vi "presets dialog.vi"(11 "Cluster in":T1={"Country 1 index"=201, "Country 2 index"=0, "countries"=[], "Data"=0, "Curve fit all data"=TRUE, "Curve 1 type"=enum."Exponential", "Curve 2 type"=enum."Exponential", "absolute?"=TRUE, "cursor 1 "=0.0, "cursor 2 "=0.0, "threshold cases"=1} {"Data" items=["cumulative cases", "new cases per day", "deaths"]}) -> (2 "Load?":bool, 3 "Cluster out":T1={"Country 1 index"=201, "Country 2 index"=0, "countries"=[], "Data"=0, "Curve fit all data"=TRUE, "Curve 1 type"=enum."Exponential", "Curve 2 type"=enum."Exponential", "absolute?"=TRUE, "cursor 1 "=0.0, "cursor 2 "=0.0, "threshold cases"=1} {"Data" items=["cumulative cases", "new cases per day", "deaths"]})   [LabVIEW 2019]
uses:
  <vilib>/Utility/sysdir.llb/System Directory Type.ctl
  <vilib>/Utility/config.llb/Write Key (I32).vi
  <vilib>/Utility/config.llb/Write Key (Boolean).vi
  <vilib>/Utility/config.llb/Write Key (Double).vi
  <vilib>/Utility/config.llb/Read Key (I32).vi
  <vilib>/Utility/config.llb/Read Key (Boolean).vi
  <vilib>/Utility/config.llb/Read Key (Double).vi
  <vilib>/Utility/config.llb/NI_LVConfig.lvlib
panel:
  in  "Delete":bool
  in  "Load":bool
  in  "Save Button":bool
  in  "Cancel Button":bool
  in  "Presets":i32(listbox)
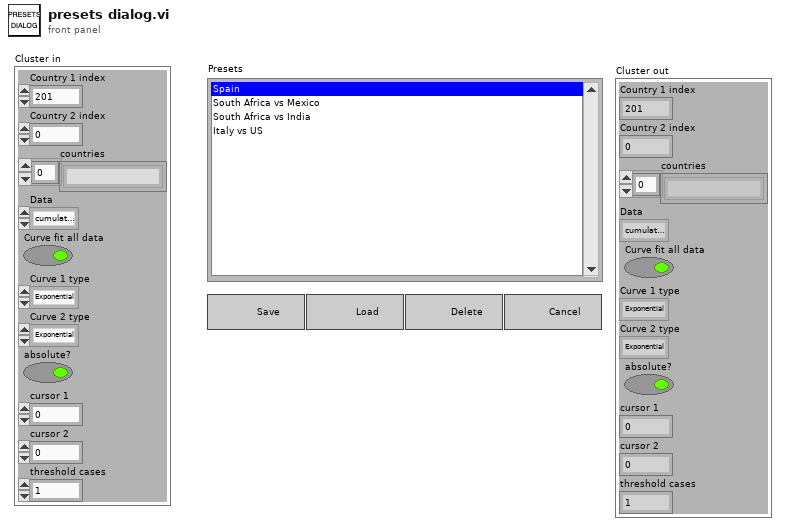
[diagram p1: front panel]
types:
  T1 = cluster{"Country 1 index":i32, "Country 2 index":i32, "countries":string[], "Data":u16, "Curve fit all data":bool, "Curve 1 type":enum16{"Exponential", "Logarithm", "No curve"}, "Curve 2 type":enum16{"Exponential", "Logarithm", "No curve"}, "absolute?":bool, "cursor 1 ":dbl, "cursor 2 ":dbl, "threshold cases":u32}
  T2 = typedef "System Directory Type.ctl" = i32
  T3 = typedef "NI_LVConfig.lvlib/Config Data RefNum.ctl" = refnum<k1>
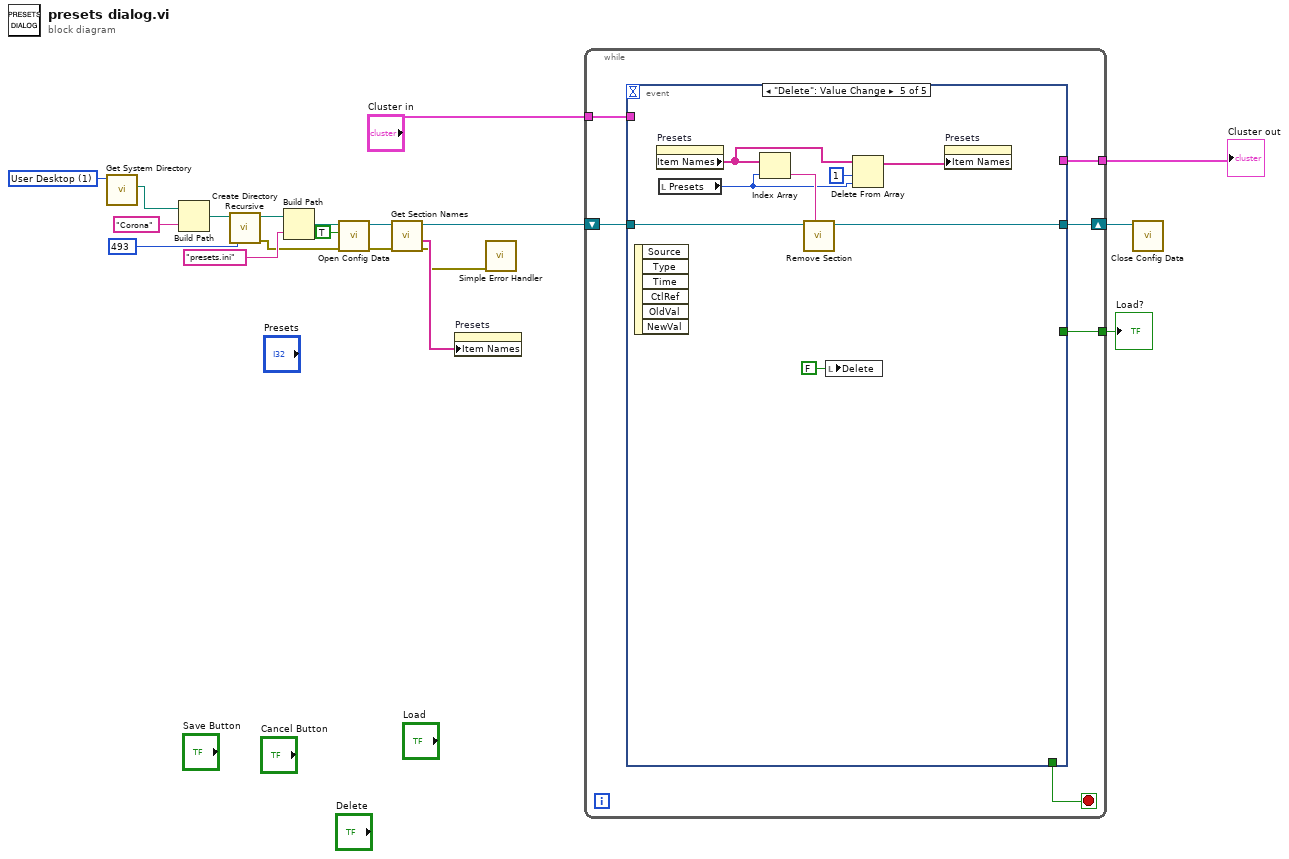
[diagram p0: block diagram]
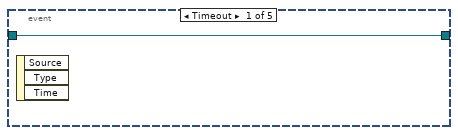
[diagram p2: hidden frame]
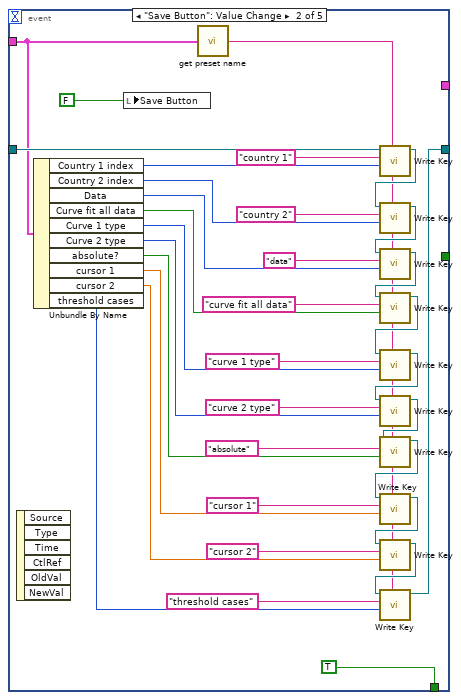
[diagram p3: hidden frame]
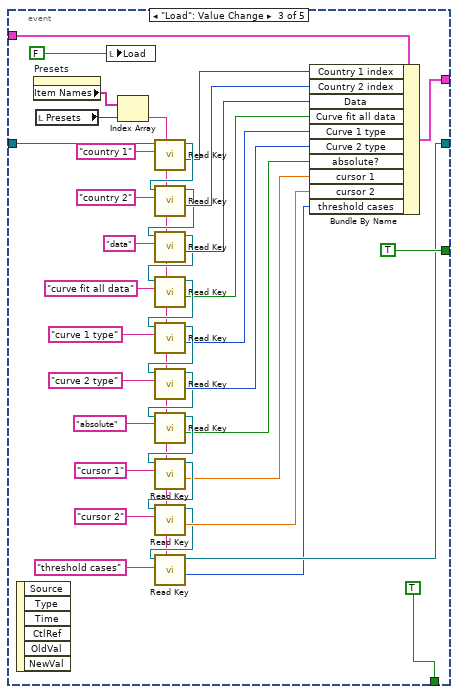
[diagram p4: hidden frame]
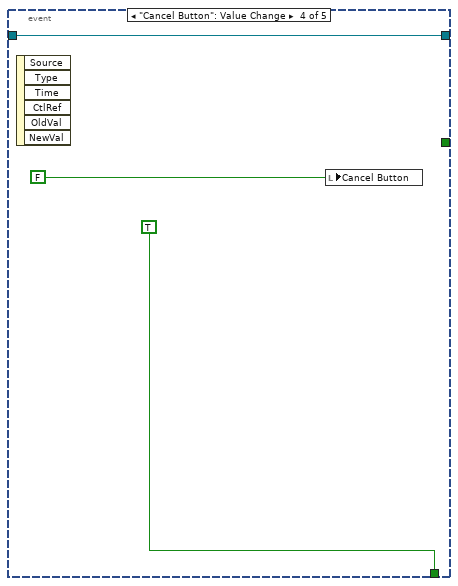
[diagram p5: hidden frame]
diagram:
  w19 = T2 1 items=["User Home"=0, "User Desktop"=1, "User Documents"=2, "User Application Data"=3, "User Preferences"=4, "User Temporary"=5, "Public Documents"=6, "Public Application Data"=7, "Public Preferences"=8, "Public Cache"=13, "System Core Libraries"=9, "System Installed Libraries"=10, "Application Files"=11, "Boot Volume Root"=12] ("system directory type")
  n1 = call <vilib>:"Get System Directory.vi"("system directory type"=w19) -> ("system directory"=w18:path)  [unwired: 10 in]
  n2 = Build Path(base path=w18, name or relative path="Corona") -> (appended path=w7:path)
  n3 = call <vilib>:"Create Directory Recursive.vi"("permissions"=i16 493, "directory"=w7) -> ("error out"=w5:errorcluster, "directory copy"=w6:path)  [unwired: 3 in, 1 out]
  n4 = Build Path(base path=w6, name or relative path="presets.ini") -> (appended path=w15:path)
  n5 = call <vilib>:"Open Config Data.vi"("error in (no error)"=w5, "create file if necessary (T)"=TRUE, "configuration file path"=w15) -> ("error out"=w9:errorcluster, "refnum"=w13:T3)  [unwired: 6 in, 1 out]
  n6 = call <vilib>:"Get Section Names.vi"("error in (no error)"=w9, "refnum"=w13) -> ("error out"=w8:errorcluster, "section names"=w11:string[], "refnum out"=w12:T3)  [unwired: 7 in]
  n7 = property on="Presets" class="LstBox (strict)"("Item Names"=w11) -> ()  [unwired: 2 in, 2 out]
  n8 = call <vilib>:"Simple Error Handler.vi"("error in (no error)"=w8) -> ()  [unwired: 4 in, 5 out]
  n9 = while {
    shift-right: [w24] -> w10
    shift-left: w12 -> [w25]
    tunnel: "Cluster in" -> [w22]
    tunnel: [w21] -> w1
    tunnel: [w20] -> w3
    stop <- w23 stop-if-true
    n10 = event shown="[4] \"Delete\": Value Change" {
      selector: _ -> [_ _ _ _ _]
      dyn-events: _ -> [_ _ _ _ _]
      timeout: _ -> [_ _ _ _ _]
      tunnel: w25 -> [w26 w61 w100 w102 w111]
      tunnel: [w26 w31 w66 w102 w109] -> w24
      tunnel: [_ TRUE TRUE TRUE _] -> w23
      tunnel: w22 -> [_ w53 w92 _ _]
      tunnel: [_ _ w91 _ _] -> w21
      tunnel: [_ _ TRUE _ _] -> w20
      event Timeout {
        n11 = event-data() -> ()  [unwired: 1 in, 3 out]
      }
      event "Save Button": Value Change {
        n12 = event-data() -> ()  [unwired: 1 in, 6 out]
        n13 = Unbundle By Name(w53) -> ("Country 1 index"=w55:i32, "Country 2 index"=w54:i32, "Data"=w51:u16, "Curve fit all data"=w37:bool, "Curve 1 type"=w36:enum16{"Exponential", "Logarithm", "No curve"}, "Curve 2 type"=w35:enum16{"Exponential", "Logarithm", "No curve"}, "absolute?"=w34:bool, "cursor 1"=w33:dbl, "cursor 2"=w32:dbl, "threshold cases"=w29:u32)
        n14 = local write "Save Button"(FALSE ("Save Button")) -> ()
        n15 = call "get preset name.vi"("Cluster in"=w53) -> ("Preset name out"=w27:string)
        n16 = call-poly <vilib>:"Write Key.vi"("section"=w27, "value"=w55, "key"="country 1", "refnum"=w61) -> ("refnum out"=w57:T3)  [unwired: 5 in, 2 out]
        n17 = call-poly <vilib>:"Write Key.vi"("section"=w27, "value"=w54, "key"="country 2", "refnum"=w57) -> ("refnum out"=w50:T3)  [unwired: 5 in, 2 out]
        n18 = call-poly <vilib>:"Write Key.vi"("section"=w27, "value"=w51, "key"="data", "refnum"=w50) -> ("refnum out"=w49:T3)  [unwired: 5 in, 2 out]
        n19 = call-poly <vilib>:"Write Key.vi"("section"=w27, "value"=w37, "key"="curve fit all data", "refnum"=w49) -> ("refnum out"=w48:T3)  [unwired: 5 in, 2 out]
        n20 = call-poly <vilib>:"Write Key.vi"("section"=w27, "value"=w36, "key"="curve 1 type", "refnum"=w48) -> ("refnum out"=w47:T3)  [unwired: 5 in, 2 out]
        n21 = call-poly <vilib>:"Write Key.vi"("section"=w27, "value"=w35, "key"="curve 2 type", "refnum"=w47) -> ("refnum out"=w46:T3)  [unwired: 5 in, 2 out]
        n22 = call-poly <vilib>:"Write Key.vi"("section"=w27, "value"=w34, "key"="absolute", "refnum"=w46) -> ("refnum out"=w45:T3)  [unwired: 5 in, 2 out]
        n23 = call-poly <vilib>:"Write Key.vi"("section"=w27, "value"=w33, "key"="cursor 1", "refnum"=w45) -> ("refnum out"=w44:T3)  [unwired: 5 in, 2 out]
        n24 = call-poly <vilib>:"Write Key.vi"("section"=w27, "value"=w32, "key"="cursor 2", "refnum"=w44) -> ("refnum out"=w30:T3)  [unwired: 5 in, 2 out]
        n25 = call-poly <vilib>:"Write Key.vi"("section"=w27, "value"=w29, "key"="threshold cases", "refnum"=w30) -> ("refnum out"=w31:T3)  [unwired: 5 in, 2 out]
      }
      event "Load": Value Change {
        n26 = event-data() -> ()  [unwired: 1 in, 6 out]
        n27 = property on="Presets" class="LstBox (strict)"() -> ("Item Names"=w94:string[])  [unwired: 2 in, 2 out]
        n28 = local read "Presets"() -> (w93:i32)
        n29 = local write "Load"(FALSE ("Save Button")) -> ()
        n30 = Index Array(array=w94, index=w93) -> (element=w63:string)
        n31 = call-poly <vilib>:"Read Key.vi"("section"=w63, "key"="country 1", "refnum"=w100) -> ("value"=w90:i32, "refnum out"=w96:T3)  [unwired: 5 in, 2 out]
        n32 = call-poly <vilib>:"Read Key.vi"("section"=w63, "key"="country 2", "refnum"=w96) -> ("value"=w89:i32, "refnum out"=w87:T3)  [unwired: 5 in, 2 out]
        n33 = call-poly <vilib>:"Read Key.vi"("section"=w63, "key"="data", "refnum"=w87) -> ("value"=w85:i32, "refnum out"=w84:T3)  [unwired: 5 in, 2 out]
        n34 = call-poly <vilib>:"Read Key.vi"("section"=w63, "key"="curve fit all data", "refnum"=w84) -> ("value"=w80:bool, "refnum out"=w83:T3)  [unwired: 5 in, 2 out]
        n35 = call-poly <vilib>:"Read Key.vi"("section"=w63, "key"="curve 1 type", "refnum"=w83) -> ("value"=w79:i32, "refnum out"=w82:T3)  [unwired: 5 in, 2 out]
        n36 = call-poly <vilib>:"Read Key.vi"("section"=w63, "key"="curve 2 type", "refnum"=w82) -> ("value"=w78:i32, "refnum out"=w73:T3)  [unwired: 5 in, 2 out]
        n37 = call-poly <vilib>:"Read Key.vi"("section"=w63, "key"="absolute", "refnum"=w73) -> ("value"=w69:bool, "refnum out"=w74:T3)  [unwired: 5 in, 2 out]
        n38 = call-poly <vilib>:"Read Key.vi"("section"=w63, "key"="cursor 1", "refnum"=w74) -> ("value"=w68:dbl, "refnum out"=w75:T3)  [unwired: 5 in, 2 out]
        n39 = call-poly <vilib>:"Read Key.vi"("section"=w63, "key"="cursor 2", "refnum"=w75) -> ("value"=w67:dbl, "refnum out"=w65:T3)  [unwired: 5 in, 2 out]
        n40 = call-poly <vilib>:"Read Key.vi"("section"=w63, "key"="threshold cases", "refnum"=w65) -> ("value"=w62:i32, "refnum out"=w66:T3)  [unwired: 5 in, 2 out]
        n41 = Bundle By Name(cluster=w92, "Country 1 index"=w90, "Country 2 index"=w89, "Data"=w85, "Curve fit all data"=w80, "Curve 1 type"=w79, "Curve 2 type"=w78, "absolute?"=w69, "cursor 1"=w68, "cursor 2"=w67, "threshold cases"=w62) -> (w91:T1)
      }
      event "Cancel Button": Value Change {
        n42 = event-data() -> ()  [unwired: 1 in, 6 out]
        n43 = local write "Cancel Button"(FALSE ("Cancel Button")) -> ()
      }
      event "Delete": Value Change {
        n44 = event-data() -> ()  [unwired: 1 in, 6 out]
        n45 = property on="Presets" class="LstBox (strict)"() -> ("Item Names"=w108:string[])  [unwired: 2 in, 2 out]
        n46 = local read "Presets"() -> (w106:i32)
        n47 = Index Array(array=w108, index=w106) -> (element=w110:string)
        n48 = call <vilib>:"Remove Section.vi"("section"=w110, "refnum"=w111) -> ("refnum out"=w109:T3)  [unwired: 7 in, 2 out]
        n49 = local write "Delete"(FALSE ("Delete")) -> ()
        n50 = Delete From Array(array=w108, length=1, index=w106) -> (array with subset deleted=w107:string[])  [unwired: 1 out]
        n51 = property on="Presets" class="LstBox (strict)"("Item Names"=w107) -> ()  [unwired: 2 in, 2 out]
      }
    }
  }
  "Load?" <- w3
  "Cluster out" <- w1
  n52 = call <vilib>:"Close Config Data.vi"("refnum"=w10) -> ()  [unwired: 9 in, 2 out]
